vi "RegisterNchwMat_U8.vi"(8 "error in":errorcluster, 11 "Array in":u8[][][][](array[numeric])) -> (0 "error out":errorcluster, 4 "Data":u8[][][][](array[numeric]), 6 "NchwInfo":T1 {"Null" format="%.0b"})   [LabVIEW 2020, in "OpenLvVision_OpenCv.lvlib"]
uses:
  OpenLvVision_OpenCv.lvlib
  TypeDef/NchwMatInfo.ctl
  TypeDef/LvDatatype.ctl
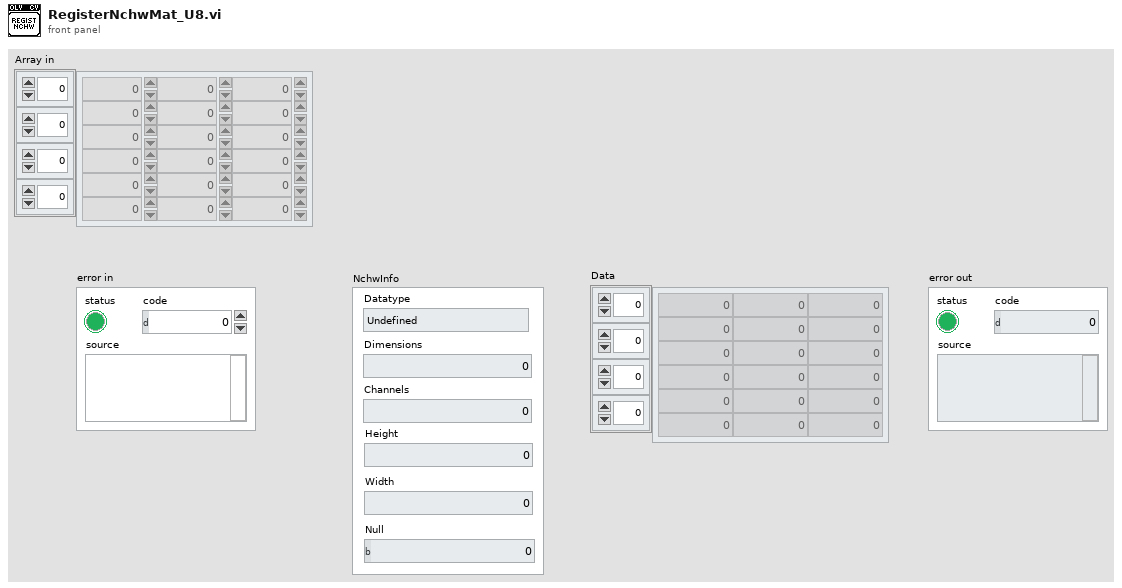
[diagram p1: front panel]
types:
  T1 = typedef "OpenLvVision_OpenCv.lvlib/NchwMatInfo.ctl" = cluster{"Datatype":T2, "Dimensions":i32, "Channels":i32, "Height":i32, "Width":i32, "Null":u8}
  T2 = typedef "OpenLvVision_OpenCv.lvlib/LvDatatype.ctl" = enum32{"Undefined", "U8", "I8", "U16", "I16", "U32_Color", "I32", "U64_Color", "I64", "SGL", "DBL", "Complex SGL", "Complex DBL", "Array 1D U8", "Array 1D I8", "Array 1D U16", "Array 1D I16", "Array 1D U32_Color", "Array 1D I32", "Array 1D U64_Color", "Array 1D I64", "Array 1D SGL", "Array 1D DBL", "Array 1D Complex SGL", "Array 1D Complex DBL", "Array 2D U8", "Array 2D I8", "Array 2D U16", "Array 2D I16", "Array 2D U32", "Array 2D U32_Color", "Array 2D I32", "Array 2D U64", "Array 2D U64_Color", "Array 2D I64", "Array 2D SGL", "Array 2D DBL", "Array 2D Complex SGL", "Array 2D Complex DBL", "Image Mono U8", "Image Mono U16", "Image Mono I16", "Image Mono SGL", "Image Color U32", "Image Color U64", "ImageComplex Sgl", "Array1d_2dPointI32", "Array1d_2dPointSGL", "Array1d_2dPointDBL", "Array1d_3dPointI32", "Array1d_3dPointSGL", "Array1d_3dPointDBL", "Array1d_4dPointI32", "Array1d_4dPointSGL", "Array1d_4dPointDBL", "ArrayNchwU8", "ArrayNchwI8", "ArrayNchwU16", "ArrayNchwI16", "ArrayNchwU32_Color", "ArrayNchwI32", "ArrayNchwU64_Color", "ArrayNchwSgl", "ArrayNchwDbl", "ArrayNchwComplexSgl", "ArrayNchwComplexDbl"}
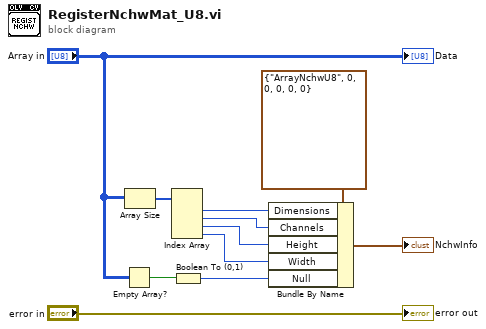
[diagram p0: block diagram]
diagram:
  n1 = Empty Array?(array="Array in") -> (empty?=w8:bool)
  n2 = Array Size(array="Array in") -> (size(s)=w5:i32[])
  n3 = Index Array(array=w5) -> (element #1=w4:i32, element #2=w3:i32, element #3=w2:i32, element #4=w1:i32)  [unwired: 4 in]
  n4 = Boolean To (0,1)(Boolean=w8) -> (0, 1=w7:i16)
  n5 = Bundle By Name(cluster=T1 {"Datatype"=enum."ArrayNchwU8", "Dimensions"=0, "Channels"=0, "Height"=0, "Width"=0, "Null"=0} ("NchwMatInfo"), "Dimensions"=w4, "Channels"=w3, "Height"=w2, "Width"=w1, "Null"=w7) -> (→"NchwInfo":T1)
  "error out" <- "error in"
  "Data" <- "Array in"
